vi "Text.vi"(4 "Position":cluster{"X":sgl, "Y":sgl, "Z":sgl}, 5 "Alpha":dbl=1.0, 6 "Path to font file":path, 7 "Color Box":u32(colorbox), 8 "error in (no error)":errorcluster, 9 "Text":string, 10 "Name":string) -> (0 "error out":errorcluster, 3 "3D Object out":refnum<class "3D Object.lvclass">)   [LabVIEW 2015, in "3D Object.lvclass"]
uses:
  3D Object.lvclass
  <vilib>/picture/3D Picture Control/NI_3D Picture Control.lvlib
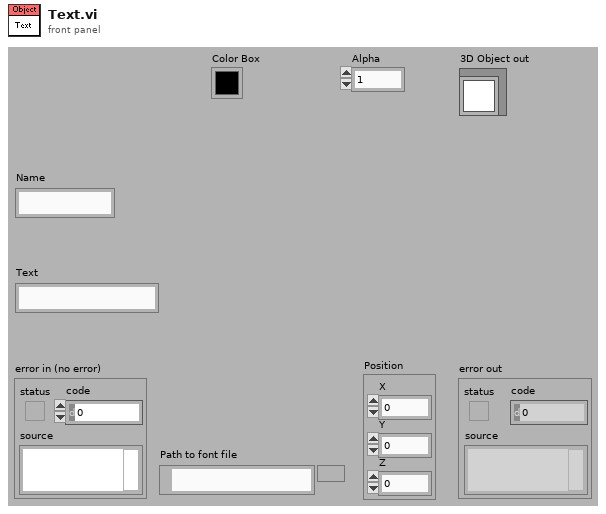
[diagram p1: front panel]
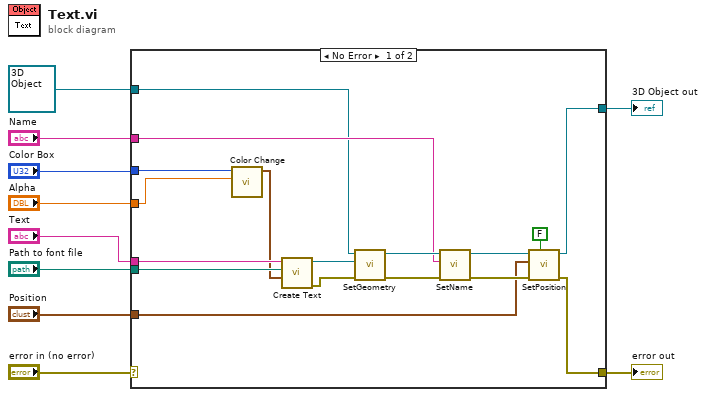
[diagram p0: block diagram]
diagram:
  n1 = case shown="No Error" "error in (no error)" {
    selector: "error in (no error)" -> [_ w29]
    tunnel: [w26 w29] -> w9
    tunnel: [w12 w28] -> w1
    tunnel: refnum<class "3D Object.lvclass"> refnum ("3D Object in") -> [w16 w28]
    tunnel: "Text" -> [w25 _]
    tunnel: "Path to font file" -> [w24 _]
    tunnel: "Color Box" -> [w22 _]
    tunnel: "Alpha" -> [w21 _]
    tunnel: "Name" -> [w17 _]
    tunnel: "Position" -> [w14 _]
    frame No Error {
      n2 = call <vilib>:"Color Change.vi"("Alpha"=w21, "Color"=w22) -> ("RGBA"=w23:cluster{"R":sgl, "G":sgl, "B":sgl, "A":sgl})  [unwired: 9 out]
      n3 = call <vilib>:"Create Text.vi"("Color"=w23, "Path to font file"=w24, "Text"=w25) -> ("error out"=w27:errorcluster, "New Text Refnum"=w11:refnum<vi>)  [unwired: 1 in, 6 out]
      n4 = call "SetGeometry.vi"("error in (no error)"=w27, "Geometry"=w11, "Object in"=w16) -> ("error out"=w15:errorcluster, "Object out"=w20:refnum<class "3D Object.lvclass">)  [unwired: 7 out]
      n5 = call "SetName.vi"("error in (no error)"=w15, "Name"=w17, "3D Object in"=w20) -> ("error out"=w18:errorcluster, "3D Object out"=w19:refnum<class "3D Object.lvclass">)  [unwired: 7 out]
      n6 = call "SetPosition.vi"("Relative?"=FALSE, "error in (no error)"=w18, "Position"=w14, "3D Object in"=w19) -> ("error out"=w26:errorcluster, "3D Object out"=w12:refnum<class "3D Object.lvclass">)  [unwired: 6 in]
    }
    frame Error {
    }
  }
  "error out" <- w9
  "3D Object out" <- w1
